vi "Query MASTER ID.vi"(7 "IP":string="192.168.23.100", 8 "error in (no error)":errorcluster) -> (0 "error out":errorcluster, 3 "MASTER DATA":T1)   [LabVIEW 2022 SP3]
uses:
  <vilib>/JDP Science/JSONtext/Next JSON Value.vi
  <vilib>/JDP Science/JSONtext/String Subset.vi
  <vilib>/JDP Science/JSONtext/Parsing/Advance past next JSON Value (inlined COPY).vi
  <vilib>/JDP Science/JSONtext/Parsing/Advance past whitespace.vi
  <vilib>/JDP Science/JSONtext/Parsing/Advance past String.vi
  <vilib>/JDP Science/JSONtext/Parsing/Advance past Number.vi
  <vilib>/JDP Science/JSONtext/Parsing/Advance past Line Ending.vi
  <vilib>/JDP Science/JSONtext/Parsing/Parse Full Path or Item Name.vi
  <vilib>/JDP Science/JSONtext/Parsing/Advance past Array.vi
  <vilib>/JDP Science/JSONtext/Parsing/Advance past Object.vi
  <vilib>/JDP Science/JSONtext/support/Error Cluster From Code.vi
  <vilib>/JDP Science/JSONtext/Offset/Find Item Locations by Path.vi
  <vilib>/httpClient/LabVIEWHTTPClient.lvlib
  <vilib>/JDP Science/JSONtext/JSONtext.lvlib
panel:
  in  "MASTER DATA INPUT CLUSTER":T1
  out "JSON data":string
  # "IO LINK Master data"
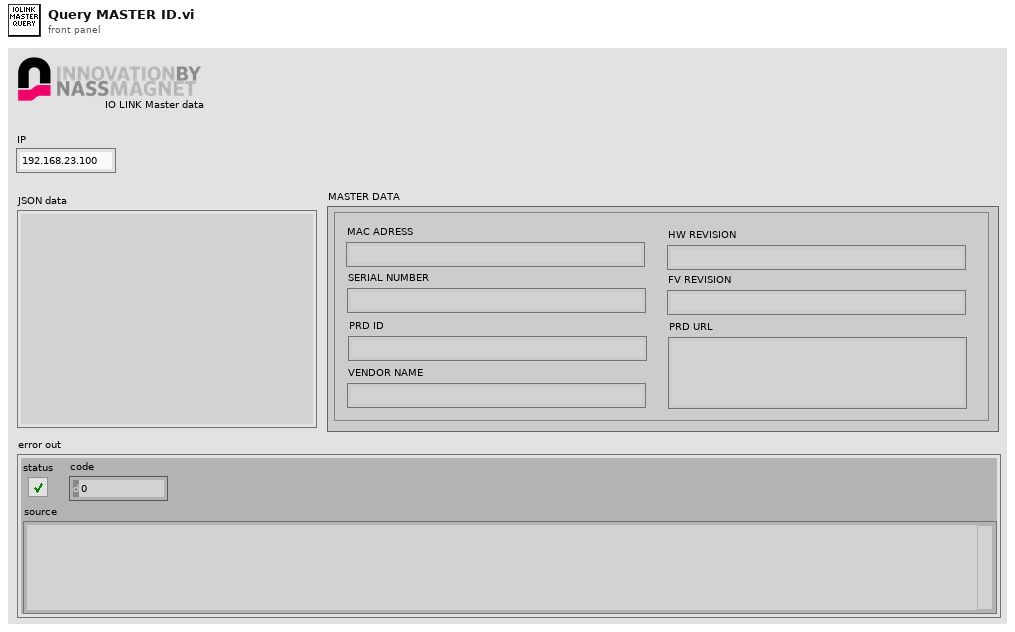
[diagram p1: front panel]
types:
  T1 = cluster{"MAC ADRESS":string, "SERIAL NUMBER":string, "PRD ID":string, "VENDOR NAME":string, "HW REVISION":string, "FV REVISION":string, "PRD URL":string}
  T2 = typedef "LabVIEWHTTPClient.lvlib/ClientHandle.ctl" = refnum<k1>
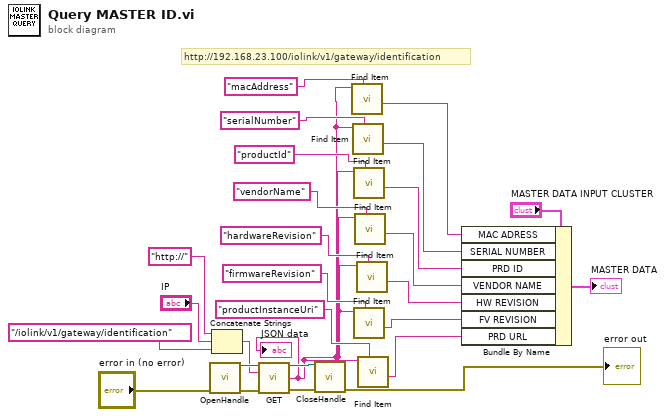
[diagram p0: block diagram]
diagram:
  # "http://192.168.23.100/iolink/v1/gateway/identification"
  n1 = call <vilib>:"OpenHandle.vi"("error in (no error)"="error in (no error)") -> ("client handle out"=w27:T2, "error out"=w26:errorcluster)  [unwired: 13 in]
  n2 = Concatenate Strings("http://" ("string"), "IP", "/iolink/v1/gateway/identification" ("string")) -> (w21:string)
  n3 = call <vilib>:"GET.vi"("client handle"=w27, "url"=w21, "error in (no error)"=w26) -> ("client handle out"=w18:T2, "body"=w11:string, "error out"=w19:errorcluster)  [unwired: 9 in, 1 out]
  "JSON data" <- w11
  n4 = call <vilib>:"CloseHandle.vi"("client handle"=w18, "error in (no error)"=w19) -> ("error out"=→"error out":errorcluster)  [unwired: 13 in]
  n5 = call <vilib>:"Find Item.vi"("$Path or Item Name"="macAddress", "JSON"=w11) -> ("<JSON>"=w8:string)  [unwired: 6 in, 3 out]
  n6 = call <vilib>:"Find Item.vi"("$Path or Item Name"="serialNumber", "JSON"=w11) -> ("<JSON>"=w7:string)  [unwired: 6 in, 3 out]
  n7 = call <vilib>:"Find Item.vi"("$Path or Item Name"="productId", "JSON"=w11) -> ("<JSON>"=w6:string)  [unwired: 6 in, 3 out]
  n8 = call <vilib>:"Find Item.vi"("$Path or Item Name"="firmwareRevision", "JSON"=w11) -> ("<JSON>"=w3:string)  [unwired: 6 in, 3 out]
  n9 = call <vilib>:"Find Item.vi"("$Path or Item Name"="vendorName", "JSON"=w11) -> ("<JSON>"=w5:string)  [unwired: 6 in, 3 out]
  n10 = call <vilib>:"Find Item.vi"("$Path or Item Name"="hardwareRevision", "JSON"=w11) -> ("<JSON>"=w4:string)  [unwired: 6 in, 3 out]
  n11 = call <vilib>:"Find Item.vi"("$Path or Item Name"="productInstanceUri", "JSON"=w11) -> ("<JSON>"=w2:string)  [unwired: 6 in, 3 out]
  n12 = Bundle By Name(cluster="MASTER DATA INPUT CLUSTER", "MAC ADRESS"=w8, "SERIAL NUMBER"=w7, "PRD ID"=w6, "VENDOR NAME"=w5, "HW REVISION"=w4, "FV REVISION"=w3, "PRD URL"=w2) -> (→"MASTER DATA":T1)
